vi "Create from Connection.vi"(7 "Manager":refnum<class "Manager.lvclass">, 8 "error in (no error)":errorcluster, 11 "Stream:Connection":refnum<class "Connection.lvclass">) -> (0 "error out":errorcluster, 3 "Endpoint out":refnum<class "Endpoint.lvclass">)   [LabVIEW 2020, in "Stream-Simple-Msg.lvlib" / "Endpoint.lvclass"]
uses:
  Endpoint.lvclass
  Manager/Manager.lvclass
  <vilib>/IlluminatedG/lv-stream/Connection/Connection.lvclass
  C:/Program Files (x86)/National Instruments/LabVIEW 2020/vi.lib/IlluminatedG/lv-stream/Endpoint/Endpoint.lvclass
  Endpoint.lvclass/Endpoint.ctl
  Read Loop Async.vi
  <vilib>/IlluminatedG/lv-stream/Endpoint/Endpoint.lvclass
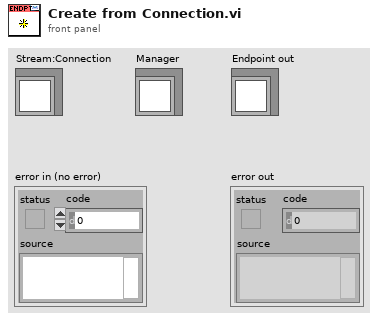
[diagram p1: front panel]
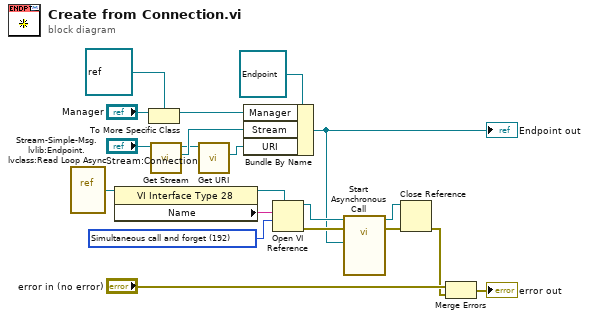
[diagram p0: block diagram]
diagram:
  w8 = 192 items=["Record modifications"=1, "Open templates for editing"=2, "Prompt user to save"=4, "Prepare for reentrant run"=8, "Prompt to find missing subVIs"=16, "Hide loading dialog box"=32, "Enable simultaneous calls"=64, "Prepare to call and forget"=128, "Simultaneous call and forget"=192, "Prepare to call and collect"=256, "Simultaneous call and collect"=320]
  n1 = vi-ref "Stream-Simple-Msg.lvlib:Endpoint.lvclass:Read Loop Async.vi"() -> (w6:refnum<vi>)
  n2 = property class="VI Interface Type 28"(reference=w6) -> (reference out=w9:refnum<vi>, "Name"=w7:string)  [unwired: 1 in, 1 out]
  n3 = To More Specific Class(target class=refnum<class> refnum ("LabVIEW Object"), reference="Manager") -> (specific class reference=w16:refnum<class>)  [unwired: 1 in, 1 out]
  n4 = call-dynamic "Get Stream.vi"("Connection in"="Stream:Connection") -> ("Stream"=w14:refnum<class "Stream.lvclass">, "Connection out"=w2:refnum<class "Connection.lvclass">)  [unwired: 8 in, 1 out]
  n5 = call <vilib>:"Get URI.vi"("Endpoint in"=w2) -> ("URI"=w1:refnum<class "URI.lvclass">)  [unwired: 8 in, 2 out]
  n6 = Bundle By Name(cluster=refnum<class "Endpoint.lvclass"> refnum ("Endpoint in"), "Manager"=w16, "Stream"=w14, "URI"=w1) -> (w5:refnum<class "Endpoint.lvclass">)
  "Endpoint out" <- w5
  n7 = Open VI Reference(type specifier VI Refnum (for type only)=w9, vi path=w7, options=w8) -> (vi reference=w11:refnum<vi>, error out=w10:errorcluster)  [unwired: 3 in]
  n8 = call-by-ref "Start Asynchronous Call"(reference=w11, error in=w10, "Endpoint in"=w5) -> (reference out=w13:refnum<vi>, error out=w12:errorcluster)  [unwired: 11 in]
  n9 = Close Reference(reference=w13, error in (no error)=w12) -> (error out=w3:errorcluster)
  n10 = Merge Errors("error in (no error)", w3) -> (→"error out":errorcluster)
